vi "Do Frame Action.vi"(8 "error in (no error)":errorcluster, 11 "Loop in":refnum<class "Loop.lvclass">) -> (0 "error out":errorcluster, 3 "Loop out":refnum<class "Loop.lvclass">)   [LabVIEW 2024, in "Ramses Sequencer.lvlib" / "Loop.lvclass"]
uses:
  Loop.lvclass
  Loop.lvclass/Loop.ctl
  Sequence/Sequence.lvclass
  Base Step/Base Step.lvclass
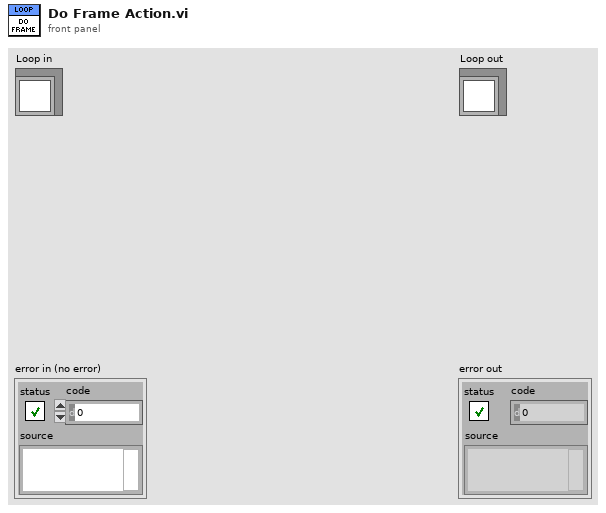
[diagram p1: front panel]
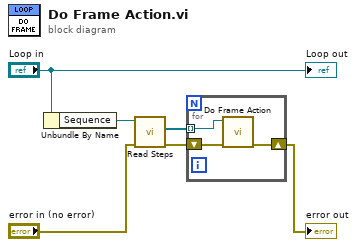
[diagram p0: block diagram]
diagram:
  n1 = Unbundle By Name("Loop in") -> ("Sequence"=w5:refnum<class "Sequence.lvclass">)
  n2 = call-dynamic "Read Steps.vi"("error in (no error)"="error in (no error)", "Sequence in"=w5) -> ("error out"=w2:errorcluster, "Steps"=w3:refnum<class "Base Step.lvclass">[])  [unwired: 7 in, 1 out]
  n3 = for {
    tunnel: w3 -> [w8] mode=indexing
    shift-right: [w7] -> w1
    shift-left: w2 -> [w9]
    n4 = call-dynamic "Do Frame Action.vi"("error in (no error)"=w9, "Base Step in"=w8) -> ("error out"=w7:errorcluster)  [unwired: 8 in, 1 out]
  }
  "error out" <- w1
  "Loop out" <- "Loop in"
